vi "计算.vi"(8 "error in (no error)":errorcluster caption="错误输入（无错误）", 11 "加法类 输入":refnum<class "加法类.lvclass"> caption="DNL_LabVIEW Object in") -> (0 "error out":errorcluster caption="错误输出", 2 "结果":dbl, 3 "加法类 输出":refnum<class "加法类.lvclass"> caption="DNL_LabVIEW Object out")   [LabVIEW 2013, in "加法类.lvclass"]
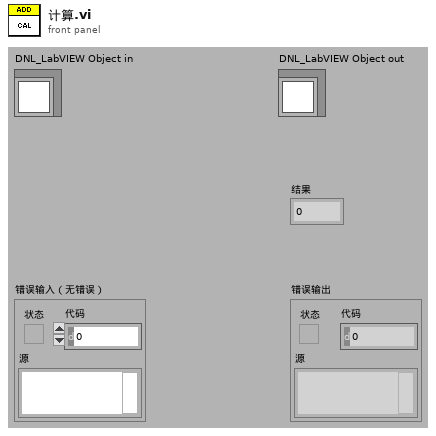
[diagram p1: front panel]
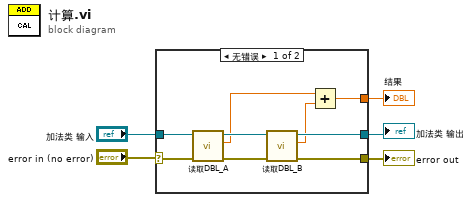
[diagram p0: block diagram]
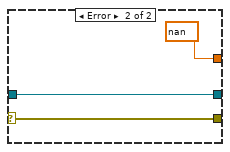
[diagram p2: hidden frame]
diagram:
  n1 = case shown="无错误" "error in (no error)" {
    selector: "error in (no error)" -> [w13 w17]
    tunnel: [w9 w17] -> w4
    tunnel: "加法类 输入" -> [w14 w16]
    tunnel: [w10 w16] -> w2
    tunnel: [w6 nan] -> w1
    frame No Error {
      n2 = call "读取DBL_A.vi"("error in (no error)"=w13, "运算类输入"=w14) -> ("error out"=w12:errorcluster, "DBL_A"=w8:dbl, "运算类输出"=w11:refnum<class "加法类.lvclass">)  [unwired: 7 in]
      n3 = call "读取DBL_B.vi"("error in (no error)"=w12, "运算类输入"=w11) -> ("error out"=w9:errorcluster, "DBL_B"=w7:dbl, "运算类输出"=w10:refnum<class "加法类.lvclass">)  [unwired: 7 in]
      n4 = Add(x=w8, y=w7) -> (x+y=w6:dbl)
    }
    frame Error {
    }
  }
  "error out" <- w4
  "加法类 输出" <- w2
  "结果" <- w1
